vi "Deadband_Filter.vi"(9 "Range":dbl=25.0 format="%#_13g", 10 "Target":dbl format="%#_13g", 11 "Joystick Input":dbl format="%#_13g") -> (3 "Output":dbl)   [LabVIEW 2016]
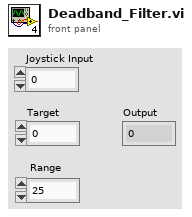
[diagram p1: front panel]
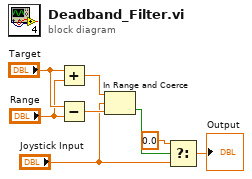
[diagram p0: block diagram]
diagram:
  n1 = Add(x="Target", y="Range") -> (x+y=w5:dbl)
  n2 = Subtract(x="Target", y="Range") -> (x-y=w4:dbl)
  n3 = In Range and Coerce(upper limit=w5, x="Joystick Input", lower limit=w4) -> (In Range?=w6:bool)  [unwired: 1 out]
  n4 = Select(t=0.0, s=w6, f="Joystick Input") -> (s? t:f=→"Output":dbl)
